vi "Add_Target.vi"(8 "Error_In":errorcluster) -> (0 "Error_Out 3":errorcluster, 3 "Target_Specification 2":T2 {"Target_Type" items=["10 Bit Address", "7 Bit Address"]})   [LabVIEW 2023]
uses:
  Controls/Menu_Ring.ctl
  Controls/Button.ctl
panel:
  in  "Add":T3
  in  "Target_Specification":T2 {"Target_Type" items=["10 Bit Address", "7 Bit Address"]}
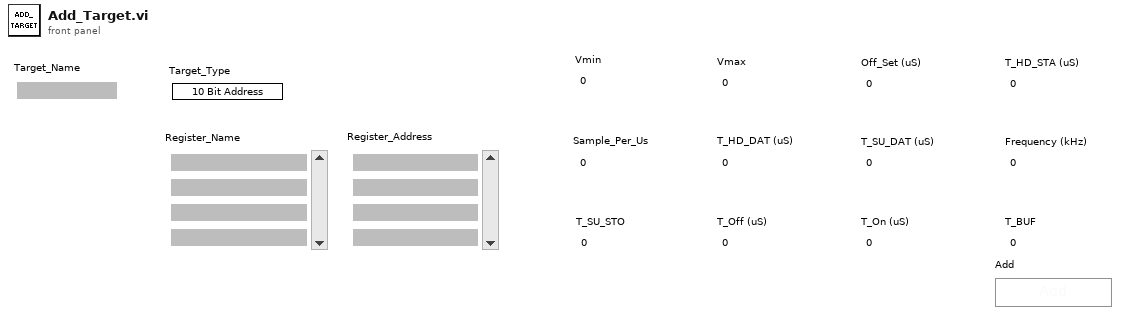
[diagram p1: front panel]
types:
  T1 = typedef "Menu_Ring.ctl" = u16
  T2 = cluster{"Target_Name":string, "Register_Name":string[], "Register_Address":string[], "Vmin":dbl, "Vmax":dbl, "Off_Set (uS)":dbl, "T_HD_STA (uS)":dbl, "T_HD_DAT (uS)":dbl, "T_SU_DAT (uS)":dbl, "Frequency (kHz)":dbl, "T_SU_STO":dbl, "T_Off (uS)":dbl, "T_On (uS)":dbl, "T_BUF":dbl, "Sample_Per_Us":dbl, "Target_Type":T1}
  T3 = typedef "Button.ctl" = bool
  T4 = enum32{"Invalid", "Standard", "Closed", "Hidden", "Minimized", "Maximized"}
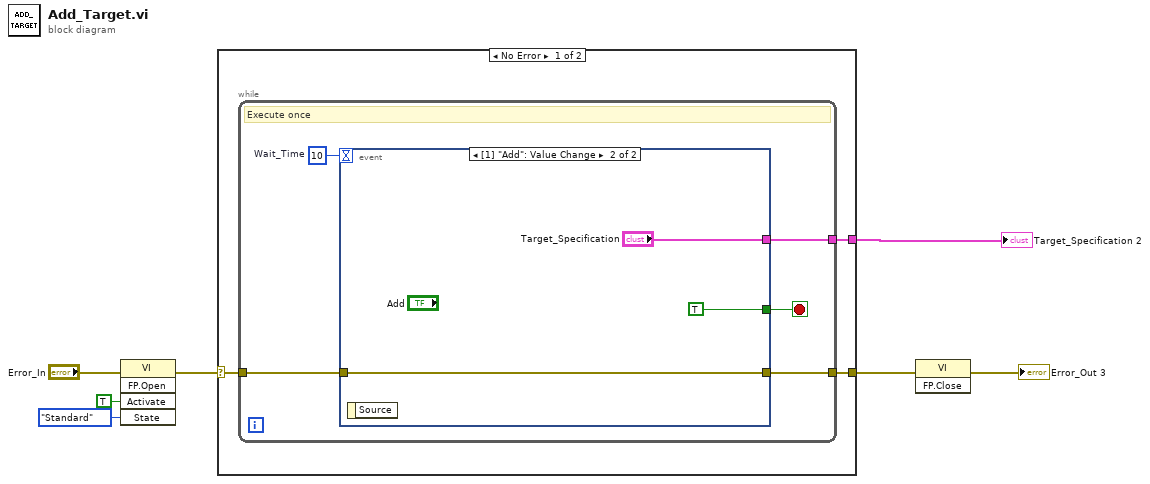
[diagram p0: block diagram]
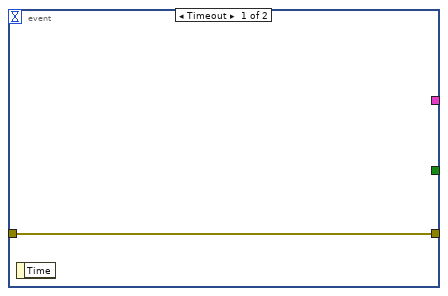
[diagram p2: hidden frame]
diagram:
  n1 = invoke class="VI" method="FP.Open"(error in="Error_In", "Activate"=TRUE ("Activate?"), "State"=T4."Standard") -> (error out=w4:errorcluster)  [unwired: 2 in, 4 out]
  n2 = case shown="No Error" w4 {
    selector: w4 -> [w9 w20]
    tunnel: [w10 _] -> w7
    tunnel: [w8 w20] -> w5
    frame No Error {
      n3 = while {
        tunnel: [w15] -> w10
        tunnel: w9 -> [w12]
        tunnel: [w11] -> w8
        stop <- w14 stop-if-true
        w13 = 10  # Wait_Time
        # "Execute once"
        n4 = event shown="[1] \"Add\": Value Change" {
          selector: _ -> [_ _]
          dyn-events: _ -> [_ _]
          timeout: w13 -> [_ _]
          tunnel: [_ "Target_Specification"] -> w15
          tunnel: [_ TRUE] -> w14
          tunnel: w12 -> [w16 w17]
          tunnel: [w16 w17] -> w11
          event Timeout {
            n5 = event-data() -> ()  [unwired: 1 in, 1 out]
          }
          event Value Change {
            n6 = event-data() -> ()  [unwired: 1 in, 1 out]
          }
        }
      }
    }
    frame Error {
    }
  }
  "Target_Specification 2" <- w7
  n7 = invoke class="VI" method="FP.Close"(error in=w5) -> (error out=→"Error_Out 3":errorcluster)  [unwired: 2 in, 2 out]
